vi "set_config_cluster.vi"(8 "error in (no error)":errorcluster, 10 "config cluster variant":variant, 11 "GenericPlugin in":refnum<class "ComponentTemplate.lvclass">) -> (0 "error out":errorcluster, 3 "GenericPlugin out":refnum<class "ComponentTemplate.lvclass">)   [LabVIEW 2010]
uses:
  ComponentTemplate.lvclass
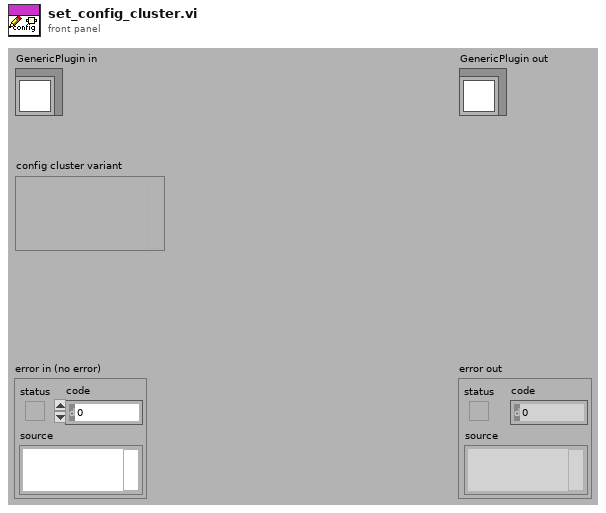
[diagram p1: front panel]
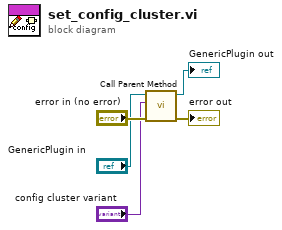
[diagram p0: block diagram]
diagram:
  n1 = call-parent "Call Parent Method"("error in (no error)"="error in (no error)", "config cluster variant"="config cluster variant", "GenericComponent in"="GenericPlugin in") -> ("error out"=→"error out":errorcluster, "GenericComponent out"=→"GenericPlugin out":refnum<class "ComponentTemplate.lvclass">)  [unwired: 7 in]
